vi "currentIndex.vi"(8 "error in (no error)":errorcluster, 11 "ScriptEditorV2 in":refnum<class "ScriptEditorV2.lvclass">) -> (0 "error out":errorcluster, 2 "index":i32, 3 "ScriptEditorV2 out":refnum<class "ScriptEditorV2.lvclass">)   [LabVIEW 2011, in "Views.lvlib" / "ScriptEditor.lvlib" / "ScriptEditorV2.lvclass"]
uses:
  ScriptEditorV2.lvclass
  ScriptEditorV2.lvclass/ScriptEditorV2.ctl
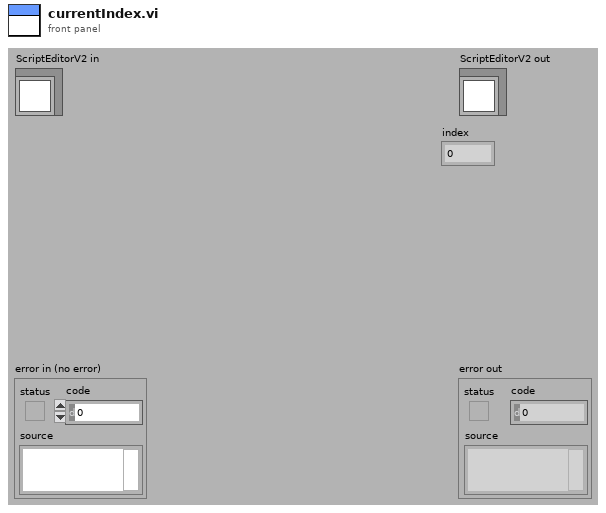
[diagram p1: front panel]
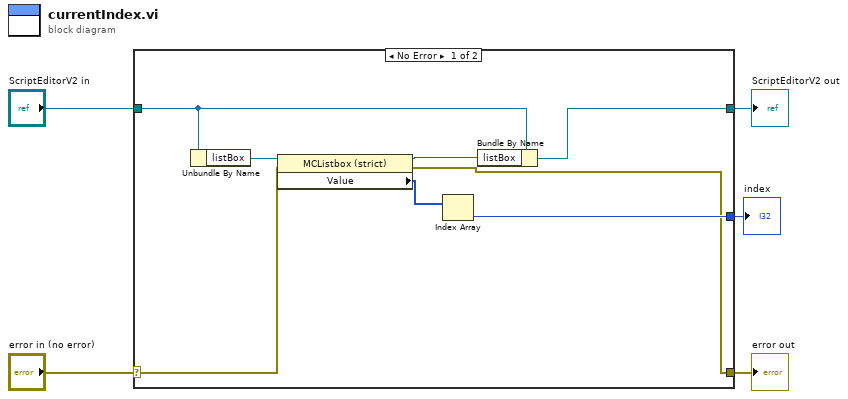
[diagram p0: block diagram]
diagram:
  n1 = case shown="No Error" "error in (no error)" {
    selector: "error in (no error)" -> [w12 w15]
    tunnel: [w6 w15] -> w4
    tunnel: [w7 w14] -> w2
    tunnel: "ScriptEditorV2 in" -> [w8 w14]
    tunnel: [w10 _] -> w1
    frame No Error {
      n2 = Unbundle By Name(w8) -> ("listBox"=w13:refnum<vi>)
      n3 = property class="MCListbox (strict)"(reference=w13, error in=w12) -> (reference out=w9:refnum<vi>, error out=w6:errorcluster, "Value"=w11:i32[])
      n4 = Index Array(array=w11) -> (element=w10:i32)  [unwired: 1 in]
      n5 = Bundle By Name(cluster=w8, "listBox"=w9) -> (w7:refnum<class "ScriptEditorV2.lvclass">)
    }
    frame Error {
    }
  }
  "error out" <- w4
  "ScriptEditorV2 out" <- w2
  "index" <- w1
